vi "2100_Test_Set State_Measure Resistance.vi"(0 "Semiconductor Module Context":T7, 1 "USID":T4 max=15, 2 "Publishable IDs":string[](array[string])=["State00", "State01", "State02", "State04", "State08"], 5 "Script_Info":T3={"Script Name"="WalkingState", "All_Scripts"=[]}, 7 "Current  Level":dbl=0.01, 9 "Instrument_Pins":T6={"SMU_Pins"=["RF1", "RF2", "RF3", "RF4"], "HSDIO_Pins"=["CLK", "SDA"]}, 11 "Error In":errorcluster, 12 "Master_Register_Data_Array_In":T1 {"Address" format="%.0x"}, 13 "Reg_Map_and_Bit_Name":T5={"Reg_Map_Bit_Name"="", "Reg_Map"=[["Reg Addr(0x00)", "7", "6", "5", "4", "3", "2", "1", "0"], ["0", "SPARE", "RF3_SH", "RF2_SH", "RF1_SH", "SPARE", "RF3_RFC", "RF2_RFC", "RF1_RFC"], ["1", "SPARE[7:0]", "", "", "", "", "", "", ""], ["2", "VVAR_EN", "LCM_EN", "RFC_SH", "SPARE", "VARACTOR[3:0]", "", "", ""], ["3", "SW_CTRL1_VIRTUAL[7:0]", "", "", "", "", "", "", ""], ["4", "SW_CTRL1_SWAP", "SW_CTRL1_RBSHIFT[2:0]", "", "", "SW_CTRL1_VSID[3:0]", "", "", ""], ["5", "REG_00_VIRTUAL_MASK[7:0]", "", "", "", "", "", "", ""], ["6", "LOCK_STATUS[1:0]", "", "CLK_DITHER", "FUSES_BURNED", "CLK_IDAC_CAL[3:0]", "", "", ""], ["7", "SPARE[2:0]", "", "", "ODFT_TRIM[4:0]", "", "", "", ""], ["8", "SPARE[2:0]", "", "", "HV_TRIM[4:0]", "", "", "", ""], ["9", "TEST_MUX[2:0]", "", "", "SPARE[1:0]", "", "MEMS_BG_TC[1:0]", "", "MEMSCP_RCM"], ["A", "CP_BOOST_OVRD_EN", "SPARE[2:0]", "", "", "PS_OFF_TIMER[1:0]", "", "PS_ON_TIMER[1:0]", ""], ["0", "", "", "", "", "", "", "", ""], ["D", "Reserved[1:0]", "", "WD_HI_EVENT_CNT[5:0]", "", "", "", "", ""], ["E", "VERSION_ID[7:0]", "", "", "", "", "", "", ""], ["F", "Reserved", "COUNT_200_LSB[6:0]", "", "", "", "", "", ""], ["10", "CLK_DIV2_EN", "Spare", "ODFT_EN", "HV_HYST[4:0]", "", "", "", ""], ["0", "", "", "", "", "", "", "", ""], ["12", "SHORT_FUSE", "FUSE_BURN", "STROBE_EN", "VIO_OK", "RTH[1:0]", "", "FUSE_LOAD_MAN_EN", "FUSE_LOAD"], ["13", "RR_ACK_EN", "Reserved", "ACK_POSITION[1:0]", "", "SuBUS_DRIVE_STRENGTH[3:0]", "", "", ""], ["14", "TM_IO_EN", "TM_IO_SEL", "SuBUS_OVS[1:0]", "", "Reserved[3:0]", "", "", ""], ["15", "Reserved[4:0]", "", "", "", "", "SuBUS_VERSION_PRESENT", "SuBUS_VOLTAGE", "SuBUS_FLAVOR_DEF"], ["16", "PROG_STROBE1_DUR[7:0]", "", "", "", "", "", "", ""], ["17", "PROG_STROBE0_DUR[7:0]", "", "", "", "", "", "", ""], ["18", "Reserved[2:0]", "", "", "EFUSE_SINGLE_ADDR_SEL[4:0]", "", "", "", ""], ["19", "POLL_ADR[4:0]", "", "", "", "", "POLL_BC[2:0]", "", ""], ["1A", "SOFTWARE_RESET", "Reserved[6:0]", "", "", "", "", "", ""], ["1B", "Reserved[7:0]", "", "", "", "", "", "", ""], ["1C", "PWR_MODE_1", "PWR_MODE_0", "TRIGGER_MASK[2:0]", "", "", "TRIGGER[2:0]", "", ""], ["1D", "PRODUCT_ID[7:0]", "", "", "", "", "", "", ""], ["1E", "MANUFACTURER_ID_LSB[7:0]", "", "", "", "", "", "", ""], ["1F", "MANUFACTURER_ID_MSB[3:0]", "", "", "", "USID[3:0]", "", "", ""]]}) -> (6 "Master_Register_Data_Array_Out":T1 {"Address" format="%.0x"}, 15 "Error Out":errorcluster)   [LabVIEW 2013]
uses:
  Controls/USID.ctl
  <vilib>/NI_TestStand_SemiconductorModule/NI_TestStand_Semiconductor_Module.lvlibp/PinMap/General/SemiconductorModuleContext.ctl
  Controls/Master_Reg_Data_Array.ctl
  Controls/Reg_Address_Data.ctl
  <vilib>/NI_TestStand_SemiconductorModule/NI_TestStand_Semiconductor_Module.lvlibp/PinMap/General/Publish/PublishDataDoubleFunctionalTest.vi
  <vilib>/NI_TestStand_SemiconductorModule/NI_TestStand_Semiconductor_Module.lvlibp
panel:
  out "R_Measurements":dbl[][](array[numeric])
  in  "Tab Control":enum32{"Test Info", "Instrument Settings"}(tab)
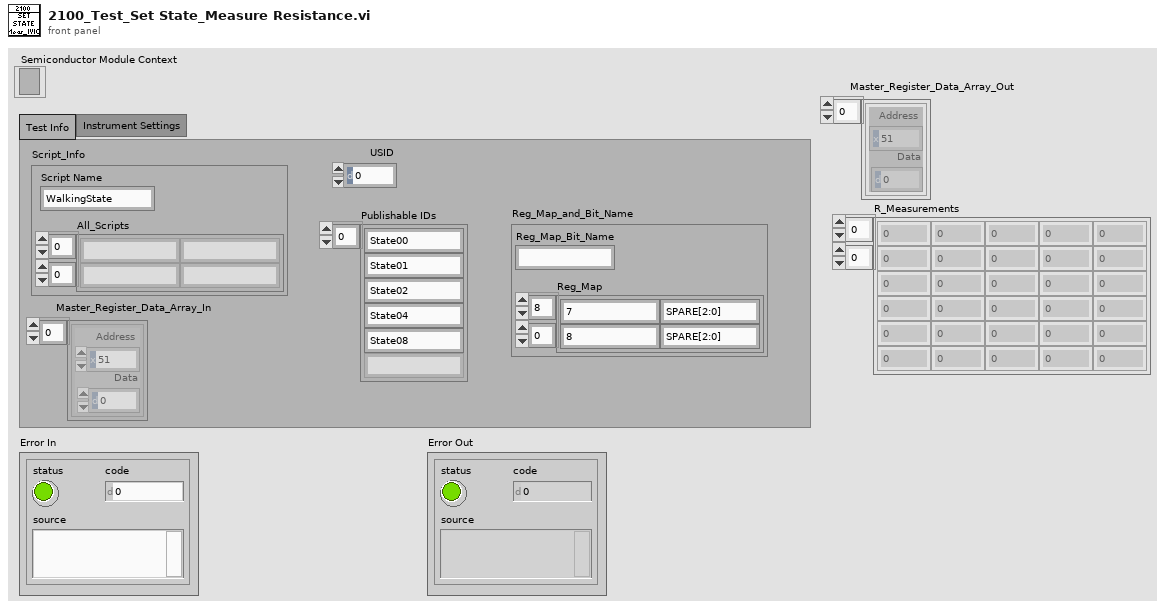
[diagram p1: front panel]
types:
  T1 = typedef "Master_Reg_Data_Array.ctl" = T2[]
  T2 = typedef "Reg_Address_Data.ctl" = cluster{"Address":u8, "Data":u8}
  T3 = cluster{"Script Name":string, "All_Scripts":string[][]}
  T4 = typedef "USID.ctl" = u8
  T5 = cluster{"Reg_Map_Bit_Name":string, "Reg_Map":string[][]}
  T6 = cluster{"SMU_Pins":string[], "HSDIO_Pins":string[]}
  T7 = typedef "NI_TestStand_Semiconductor_Module.lvlibp/SemiconductorModuleContext.ctl" = refnum<k7>
  T8 = typedef "Script Functions_Array.ctl" = enum16{"Reg_Write", "Bit_Write", "Delay", "Read", "Measure"}[]
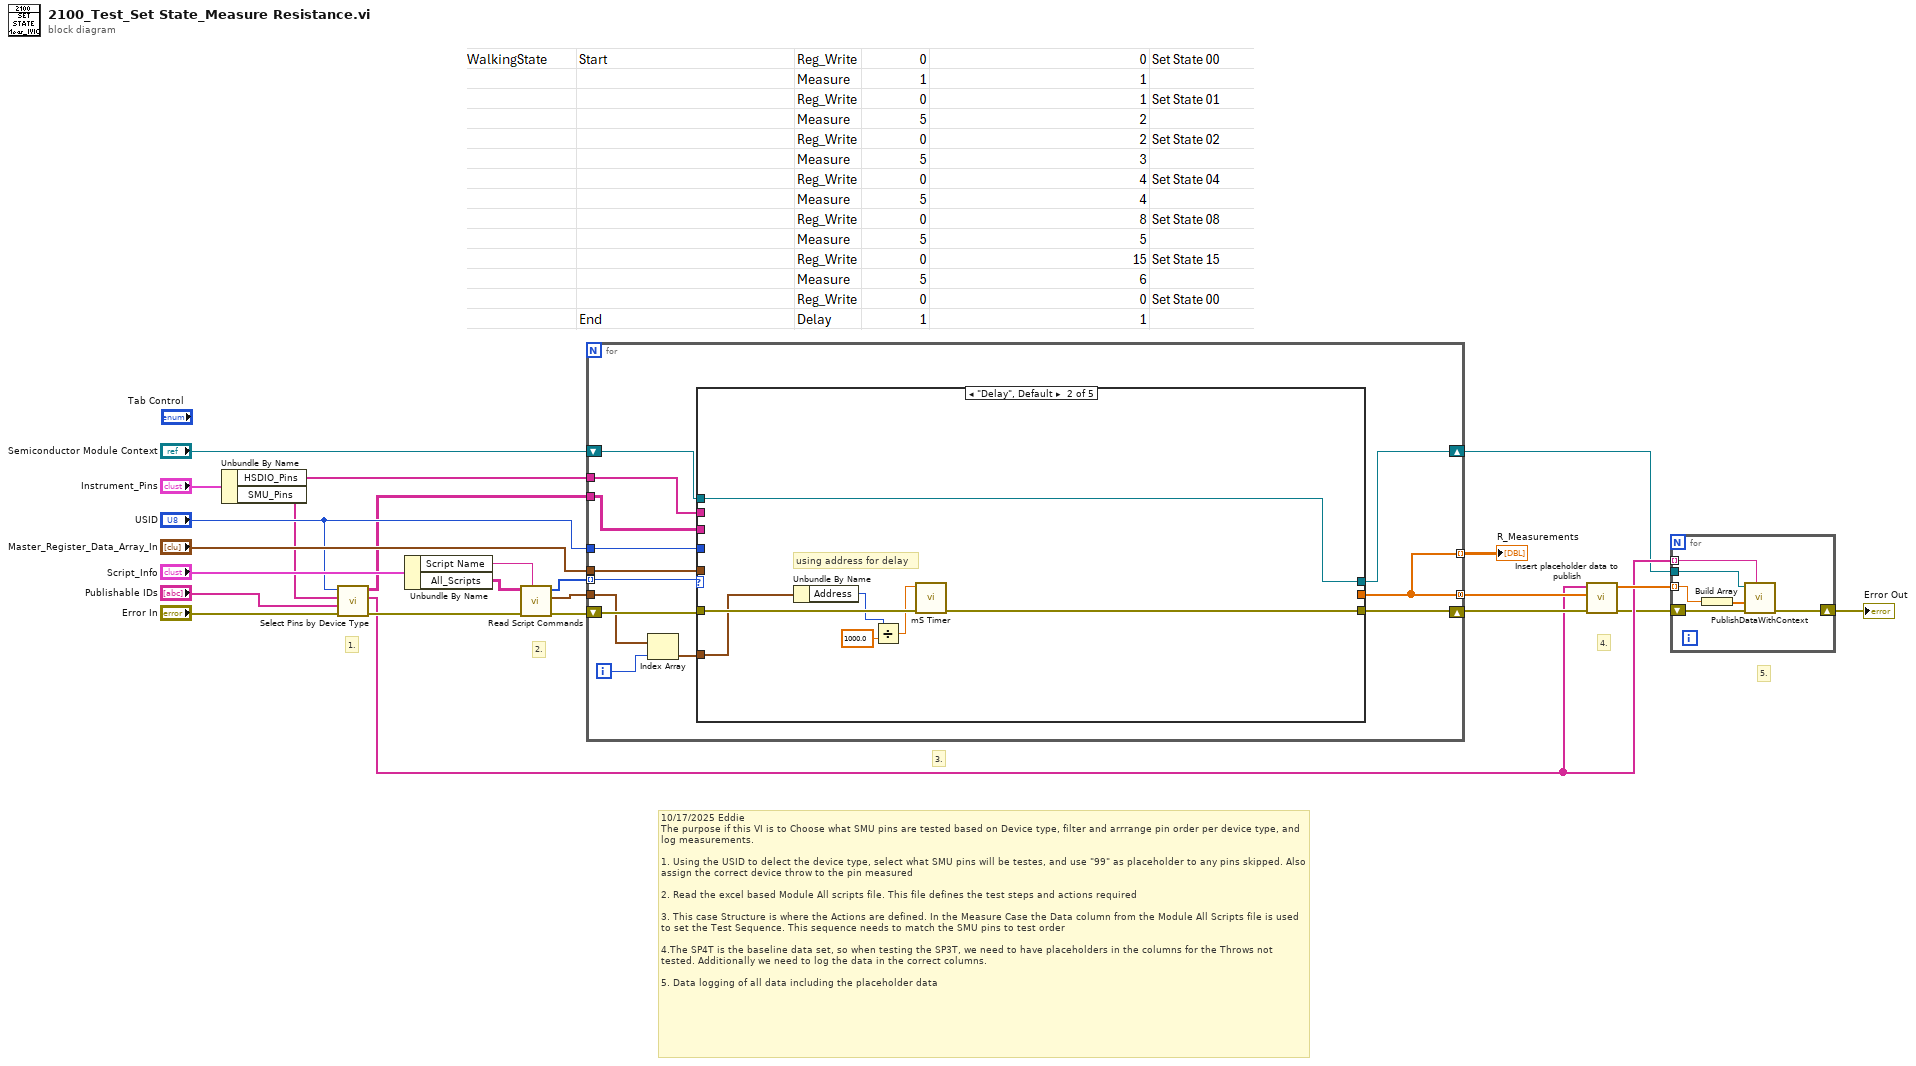
[diagram p0: block diagram]
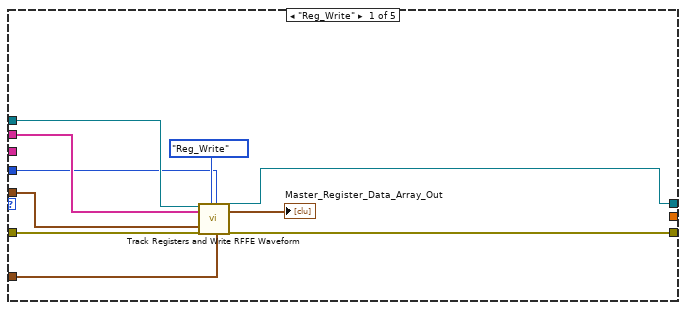
[diagram p2: hidden frame]
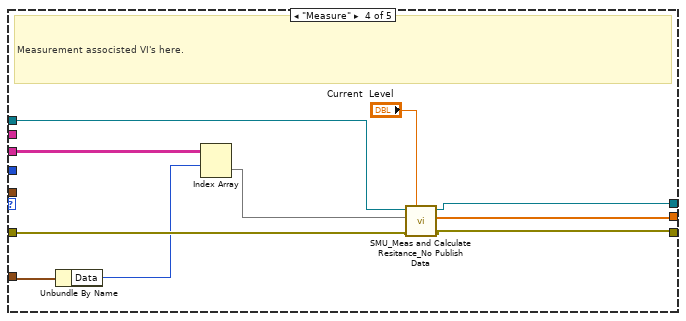
[diagram p4: hidden frame]
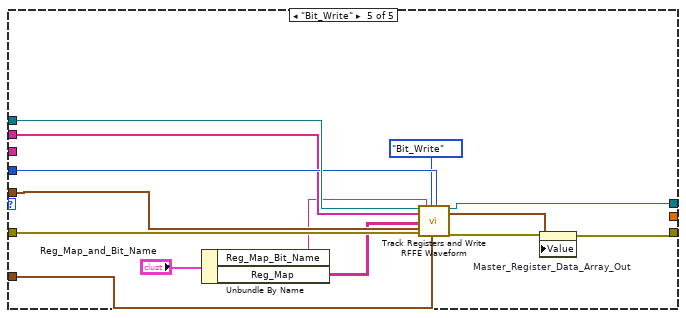
[diagram p5: hidden frame]
diagram:
  # "10/17/2025 Eddie \nThe purpose if this VI is to Choose what SMU pins are tested based on Device type, filter and arrrange pin order per device type, and log measurements.\n\n1. Using the USID to delect the device type, select what SMU pins will be testes, and use \"99\" as placeholder to any pins skipped. Also assign the correct device throw to the pin measured\n\n2. Read the excel based Module All scripts file. This file defines the test steps and actions required\n\n3. This case Structure is where the Actions are defined. In the Measure Case the Data column from the Module All Scripts file is used to set the Test Sequence. This sequence needs to match the SMU pins to test order\n\n4.The SP4T is the baseline data set, so when testing the SP3T, we need to have placeholders in the columns for the Throws not tested. Additionally we need to log the data in the correct columns.\n\n5. Data logging of all data including the placeholder data"
  # "5."
  # "4."
  # "3."
  # "2."
  # "1."
  n1 = Unbundle By Name("Instrument_Pins") -> ("HSDIO_Pins"=w17:string[], "SMU_Pins"=w10:string[])
  n2 = call "Select Pins by Device Type.vi"("error in (no error)"="Error In", "Publishable IDs"="Publishable IDs", "SP4T_Pins"=w10, "USID"="USID") -> ("error out"=w12:errorcluster, "Published ID"=w3:string[], "Pins to Test"=w9:string[][])  [unwired: 5 in]
  n3 = Unbundle By Name("Script_Info") -> ("Script Name"=w14:string, "All_Scripts"=w15:string[][])
  n4 = call "Read Script Commands.vi"("Test Name"=w14, "Error In"=w12, "All_Scripts"=w15) -> ("Error Out"=w22:errorcluster, "Script_Data"=w23:T2[], "Script_Functions"=w24:T8)  [unwired: 5 in, 1 out]
  n5 = for {
    tunnel: "USID" -> [w31]
    tunnel: w24 -> [w30] mode=indexing
    tunnel: w23 -> [w34]
    tunnel: w17 -> [w35]
    shift-right: [w28] -> w4
    shift-left: w22 -> [w37]
    tunnel: "Master_Register_Data_Array_In" -> [w32]
    tunnel: [w26] -> w20 mode=indexing
    tunnel: w9 -> [w27]
    tunnel: [w26] -> w8 mode=concatenating
    shift-right: [w25] -> w1
    shift-left: "Semiconductor Module Context" -> [w36]
    i -> [w29]
    n6 = Index Array(array=w34, index=w29) -> (element=w33:T2)
    n7 = case shown="\"Delay\", Default" w30 {
      tunnel: w33 -> [w42 w53 _ w61 w67]
      tunnel: w37 -> [w47 w54 w56 w65 w80]
      tunnel: w31 -> [w39 _ _ _ w74]
      tunnel: w36 -> [w45 w48 w55 w64 w75]
      tunnel: w35 -> [w44 _ _ _ w72]
      tunnel: [w46 w52 w56 w66 w78] -> w28
      tunnel: w32 -> [w41 _ _ _ w71]
      tunnel: [_ _ _ w62 _] -> w26
      tunnel: w27 -> [_ _ _ w60 _]
      tunnel: [w38 w48 w55 w57 w76] -> w25
      frame "Reg_Write" {
        n8 = call "Track Registers and Write RFFE Waveform.vi"("Semiconductor Module Context"=w45, "Pins"=w44, "Master_Register_Data_Array_In"=w41, "Error In"=w47, "Script_Functions"=enum16{"Reg_Write", "Bit_Write"}."Reg_Write", "USID"=w39, "Reg_Address_Data"=w42) -> ("Semiconductor Module Context Out"=w38:T7, "Master_Register_Data_Array_Out"=→"Master_Register_Data_Array_Out":T1, "Error Out"=w46:errorcluster)  [unwired: 10 in]
      }
      frame "Delay", Default {
        # "using address for delay"
        n9 = Unbundle By Name(w53) -> ("Address"=w50:u8)
        n10 = Divide(x=w50, y=1000.0) -> (x/y=w49:dbl)
        n11 = call "mS Timer.vi"("Error In"=w54, "Delay(S)"=w49) -> ("Error Out"=w52:errorcluster)  [unwired: 9 in]
      }
      frame "Read" {
        # "Future Dev Code"
      }
      frame "Measure" {
        # "Measurement associsted VI's here."
        n12 = Unbundle By Name(w61) -> ("Data"=w59:u8)
        n13 = Index Array(array=w60, index (row)=w59) -> (element=w58:string[])  [unwired: 1 in]
        n14 = call "SMU_Meas and Calculate Resitance_No Publish Data.vi"("Current  Level"="Current  Level", "error in (no error)"=w65, "Pins"=w58, "Semiconductor Module Context"=w64) -> ("error Out"=w66:errorcluster, "R Array"=w62:dbl[], "Semiconductor Module Context Out"=w57:T7)  [unwired: 5 in]
      }
      frame "Bit_Write" {
        n15 = Unbundle By Name("Reg_Map_and_Bit_Name") -> ("Reg_Map_Bit_Name"=w69:string, "Reg_Map"=w68:string[][])
        n16 = call "Track Registers and Write RFFE Waveform.vi"("Semiconductor Module Context"=w75, "Pins"=w72, "Reg_Map"=w68, "Master_Register_Data_Array_In"=w71, "Error In"=w80, "Reg_Map_Bit_Name"=w69, "Script_Functions"=enum16{"Reg_Write", "Bit_Write"}."Bit_Write", "USID"=w74, "Reg_Address_Data"=w67) -> ("Semiconductor Module Context Out"=w76:T7, "Master_Register_Data_Array_Out"=w77:T1, "Error Out"=w79:errorcluster)  [unwired: 8 in]
        n17 = property on="Master_Register_Data_Array_Out" class="Arr (strict)"(error in=w79, "Value"=w77) -> (error out=w78:errorcluster)  [unwired: 1 in, 1 out]
      }
    }
  }
  "R_Measurements" <- w20
  n18 = call "Insert placeholder data to publish .vi"("error in (no error)"=w4, "Measured_Data"=w8, "Publishable IDs"=w3) -> ("error out"=w2:errorcluster, "Array"=w7:dbl[])  [unwired: 7 in]
  n19 = for {
    tunnel: w7 -> [w83] mode=indexing
    tunnel: w3 -> [w86] mode=indexing
    shift-right: [w85] -> w5
    shift-left: w2 -> [w84]
    tunnel: w1 -> [w81]
    n20 = Build Array(w83) -> (w82:dbl[])
    n21 = call-poly <vilib>:"PublishDataWithContext.vi"("Published Data Id"=w86, "error in (no error)"=w84, "Data In"=w82, "Semiconductor Module Context"=w81) -> ("error out"=w85:errorcluster)  [unwired: 6 in, 1 out]
  }
  "Error Out" <- w5
